vi "Get Master Device Adress (SubVI).vi"(8 "entrée d'erreur (pas d'erreur)":errorcluster, 10 "DeviceKey In":string, 11 "Refnum de .NET en entrée":refnum<k24>) -> (0 "sortie d'erreur":errorcluster, 1 "DeviceKey Out":string, 2 "Device Address":i32, 3 "Refnum de .NET en sortie":refnum<k24>)   [LabVIEW 2017]
uses:
  dll/CmdLib.dll
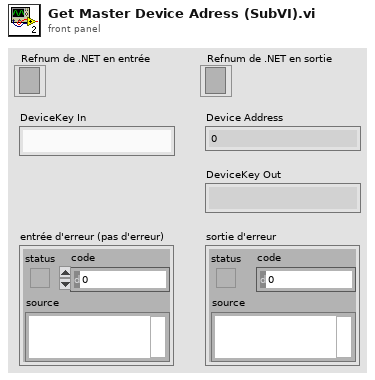
[diagram p1: front panel]
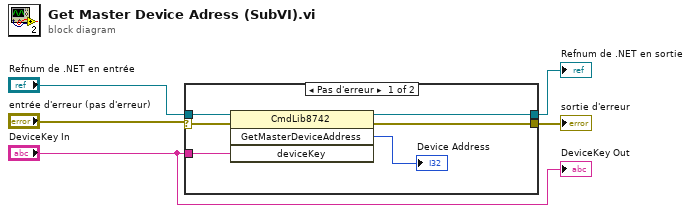
[diagram p0: block diagram]
diagram:
  n1 = case shown="Pas d'erreur" "entrée d'erreur (pas d'erreur)" {
    selector: "entrée d'erreur (pas d'erreur)" -> [w10 w13]
    tunnel: "Refnum de .NET en entrée" -> [w11 w12]
    tunnel: [w6 w12] -> w2
    tunnel: "DeviceKey In" -> [w9 _]
    tunnel: [w7 w13] -> w5
    frame No Error {
      n2 = invoke class="CmdLib8742" method="GetMasterDeviceAddress"(reference=w11, error in=w10, "deviceKey"=w9) -> (reference out=w6:refnum<k24>, error out=w7:errorcluster, "GetMasterDeviceAddress"=→"Device Address":i32)  [unwired: 1 in, 1 out]
    }
    frame Error {
    }
  }
  "Refnum de .NET en sortie" <- w2
  "sortie d'erreur" <- w5
  "DeviceKey Out" <- "DeviceKey In"
